vi "雷达流速仪读数据.vi"(6 "Error in":errorcluster caption="Error in (no error)") -> (0 "error out":errorcluster, 2 "采集数据":sgl[](array[numeric]))   [LabVIEW 2016, in "雷达流速仪.lvlib"]
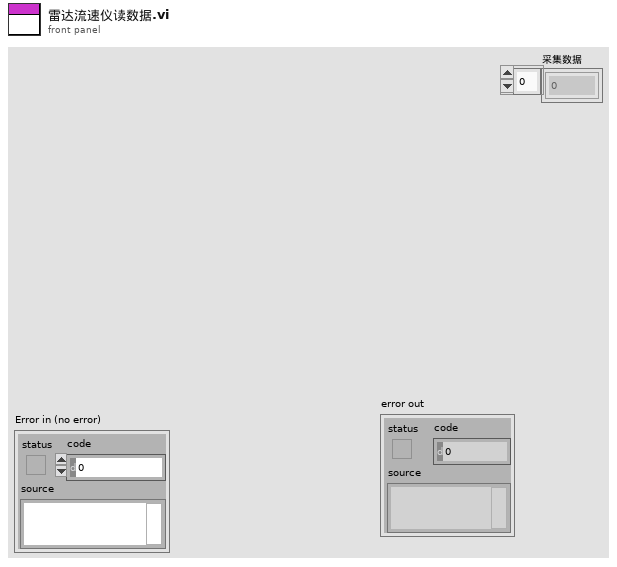
[diagram p1: front panel]
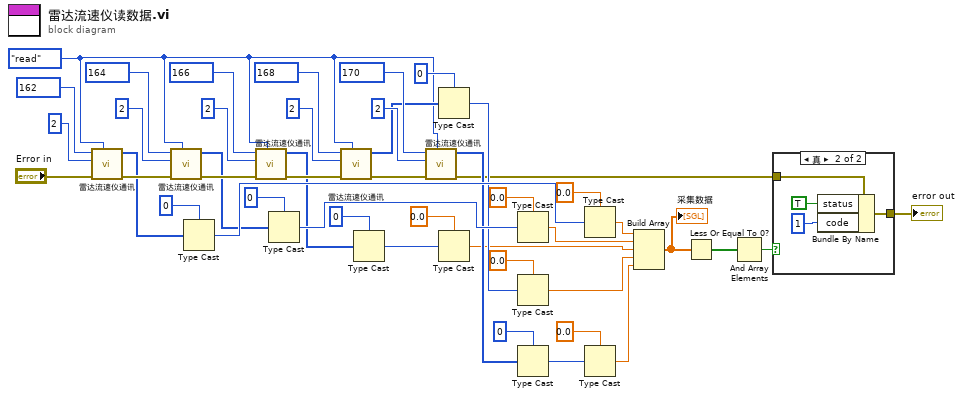
[diagram p0: block diagram]
diagram:
  w7 = enum16{"open", "read", "write", "close"}."read" ("STEP")
  n1 = call "雷达流速仪通讯.vi"("STEP"=w7, "Error in"="Error in", "quantity"=u16 2, "starting address"=u16 162) -> ("error out"=w36:errorcluster, "Registers"=w29:u16[])  [unwired: 5 in, 1 out]
  n2 = call "雷达流速仪通讯.vi"("STEP"=w7, "Error in"=w36, "quantity"=u16 2, "starting address"=u16 164) -> ("error out"=w37:errorcluster, "Registers"=w25:u16[])  [unwired: 5 in, 1 out]
  n3 = Type Cast(type=u64 0, x=w29) -> (*(type *) &x=w30:u64)
  n4 = call "雷达流速仪通讯.vi"("STEP"=w7, "Error in"=w37, "quantity"=u16 2, "starting address"=u16 166) -> ("error out"=w38:errorcluster, "Registers"=w21:u16[])  [unwired: 5 in, 1 out]
  n5 = Type Cast(type=u64 0, x=w25) -> (*(type *) &x=w28:u64)
  n6 = call "雷达流速仪通讯.vi"("STEP"=w7, "Error in"=w38, "quantity"=u16 2, "starting address"=u16 168) -> ("error out"=w33:errorcluster, "Registers"=w17:u16[])  [unwired: 5 in, 1 out]
  n7 = Type Cast(type=u64 0, x=w21) -> (*(type *) &x=w22:u64)
  n8 = call "雷达流速仪通讯.vi"("STEP"=w7, "Error in"=w33, "quantity"=u16 2, "starting address"=u16 170) -> ("error out"=w2:errorcluster, "Registers"=w13:u16[])  [unwired: 5 in, 1 out]
  n9 = Type Cast(type=u64 0, x=w17) -> (*(type *) &x=w20:u64)
  n10 = Type Cast(type=sgl 0.0, x=w22) -> (*(type *) &x=w10:sgl)
  n11 = Type Cast(type=sgl 0.0, x=w28) -> (*(type *) &x=w11:sgl)
  n12 = Type Cast(type=sgl 0.0, x=w20) -> (*(type *) &x=w9:sgl)
  n13 = Type Cast(type=u64 0, x=w13) -> (*(type *) &x=w14:u64)
  n14 = Type Cast(type=sgl 0.0, x=w30) -> (*(type *) &x=w12:sgl)
  n15 = Type Cast(type=sgl 0.0, x=w14) -> (*(type *) &x=w8:sgl)
  n16 = Build Array(w12, w11, w10, w9, w8) -> (w5:sgl[])
  "采集数据" <- w5
  n17 = Less Or Equal To 0?(x=w5) -> (x <= 0?=w4:bool[])
  n18 = And Array Elements(Boolean array=w4) -> (logical AND=w3:bool)
  n19 = case shown="真" w3 {
    tunnel: w2 -> [w47 w51]
    tunnel: [w47 w49] -> w1
    frame False {
    }
    frame True {
      n20 = Bundle By Name(cluster=w51, "status"=TRUE, "code"=1) -> (w49:errorcluster)
    }
  }
  "error out" <- w1
